vi "exercice4-1.vi"() -> ()   [LabVIEW 2013]
panel:
  out "Moyenne Deroulant":dbl
  out "Historique  Temperature":cluster{"temeperature":dbl, dbl}(graph)
  in  "Stop":bool=TRUE
  # "Marche"
  # "Arret"
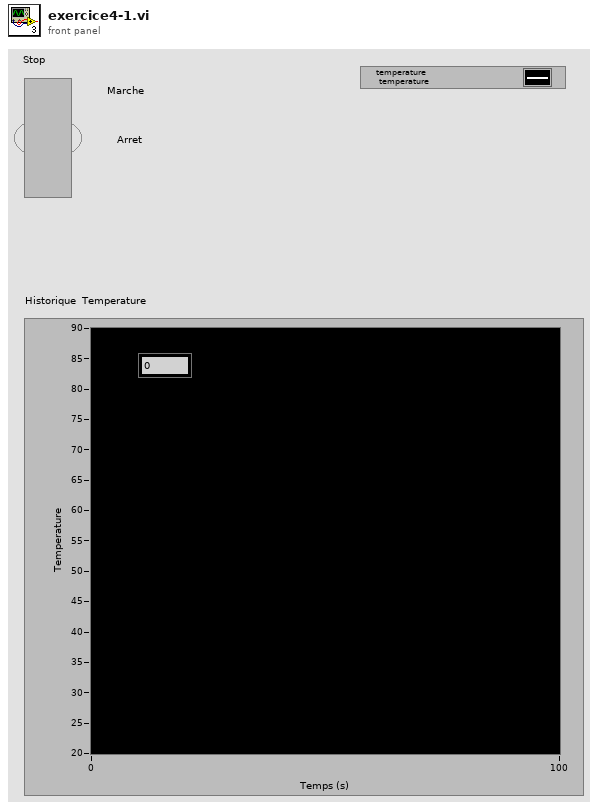
[diagram p1: front panel]
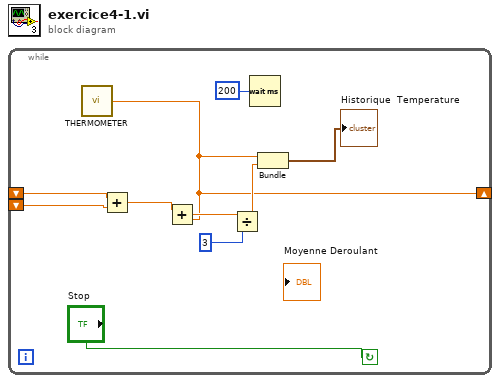
[diagram p0: block diagram]
diagram:
  n1 = while {
    shift-right: [w2] -> _
    shift-left: _ -> [w5]
    shift-left: _ -> [w4]
    stop <- "Stop" continue-if-true
    n2 = call "THERMOMETER.vi"() -> ("temeperature"=w2:dbl)  [unwired: 1 in]
    n3 = Add(x=w5, y=w4) -> (x+y=w10:dbl)
    n4 = Add(x=w10, y=w2) -> (x+y=w9:dbl)
    n5 = Divide(x=w9, y=3) -> (x/y=w3:dbl)
    n6 = Wait (ms)(milliseconds to wait=200) -> ()  [unwired: 1 out]
    n7 = Bundle("temeperature"=w2, w3) -> (→"Historique  Temperature":cluster{"temeperature":dbl, dbl})  [unwired: 1 in]
  }
